vi "Set-control-enable-multiple.vi"(8 "error in (no error)":errorcluster, 9 "Enable?":bool, 10 "Control names":T1[](array[typedef]), 11 "Panes in":T2) -> (0 "error out":errorcluster, 3 "Panes out":T2)   [LabVIEW 2013, in "HardwareCharacterization.lvlib" / "HC-UI.lvclass"]
uses:
  HC-UI.lvclass
  Panes-reference.ctl
  Control-names.ctl
  HC-UI.lvclass/HC-UI.ctl
  Read Controls lib.vi
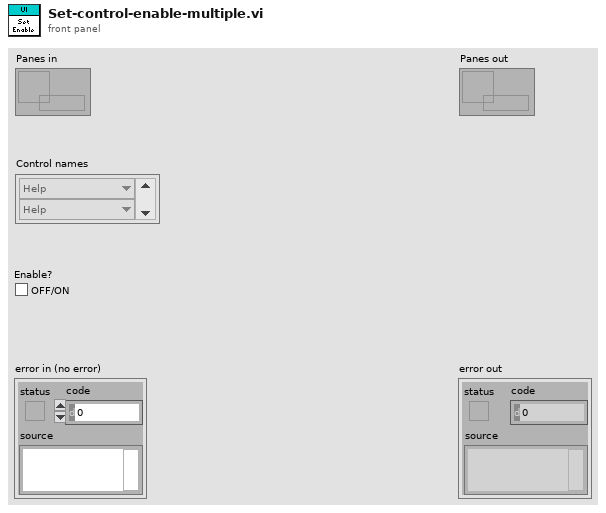
[diagram p1: front panel]
types:
  T1 = typedef "HardwareCharacterization.lvlib/HC-UI.lvclass/Control-names.ctl" = enum16{"Help", "Status", "Load configuration", "Save configuration", "Activate", "Start", "Stop", "Options"}
  T2 = typedef "HardwareCharacterization.lvlib/HC-UI.lvclass/Panes-reference.ctl" = refnum<data-value>
  T3 = enum8{"Enabled", "Disabled", "Disabled and Grayed Out"}
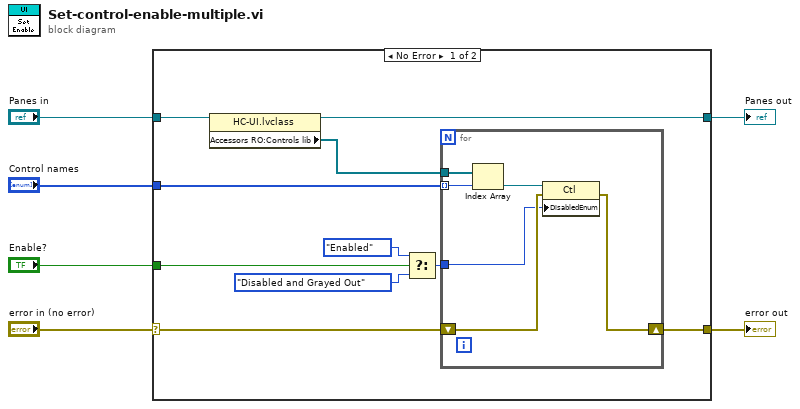
[diagram p0: block diagram]
diagram:
  n1 = case shown="No Error" "error in (no error)" {
    selector: "error in (no error)" -> [w11 w23]
    tunnel: [w13 w23] -> w5
    tunnel: [w12 w24] -> w3
    tunnel: "Panes in" -> [w16 w24]
    tunnel: "Control names" -> [w14 _]
    tunnel: "Enable?" -> [w10 _]
    frame No Error {
      n2 = property class="HC-UI.lvclass"(reference=w16) -> (reference out=w12:T2, "Accessors RO:Controls lib"=w15:refnum<vi>[])  [unwired: 1 in, 1 out]
      n3 = Select(t=T3."Enabled" ("Disabled"), s=w10, f=T3."Disabled and Grayed Out" ("Disabled")) -> (s? t:f=w9:T3)
      n4 = for {
        tunnel: w15 -> [w22]
        tunnel: w14 -> [w21] mode=indexing
        tunnel: w9 -> [w17]
        shift-right: [w20] -> w13
        shift-left: w11 -> [w18]
        n5 = Index Array(array=w22, index=w21) -> (element=w19:refnum<vi>)
        n6 = property class="Ctl"(reference=w19, error in=w18, "DisabledEnum"=w17) -> (error out=w20:errorcluster)  [unwired: 1 out]
      }
    }
    frame Error {
    }
  }
  "error out" <- w5
  "Panes out" <- w3
